vi "CCD Example.vi"(0 "exposure time [ms]":i32=120, 9 "roiConfig":T1={"ROI-index"=1, "xOrigin"=0, "yOrigin"=0, "xSize"=1024, "ySize"=256, "xBin"=1, "yBin"=256}, 11 "error in":errorcluster) -> (4 "ExposureTime [ms]":i32, 6 "device is open?":bool, 13 "chip size, x":i32, 14 "chip size, y":i32, 15 "error out":errorcluster)   [LabVIEW 2023, in "Examples.lvlib"]
doc: "Example for a CCD spectrum acquisition."
uses:
  Examples.lvlib
  Classes/CCD/CCD.lvclass
panel:
  # "Connector Pane"
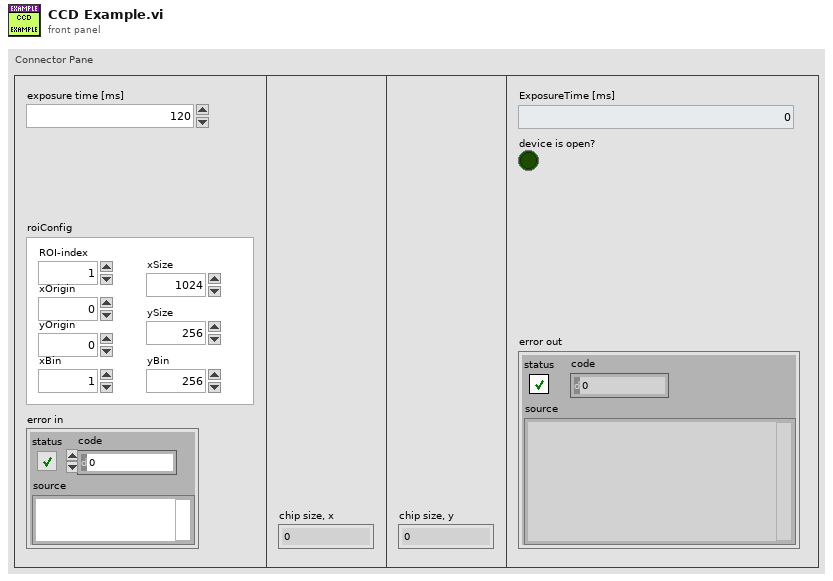
[diagram p1: front panel]
types:
  T1 = cluster{"ROI-index":i32, "xOrigin":i32, "yOrigin":i32, "xSize":i32, "ySize":i32, "xBin":i32, "yBin":i32}
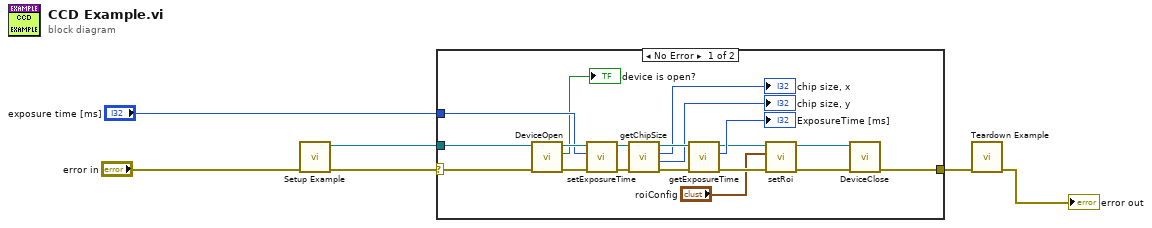
[diagram p0: block diagram]
diagram:
  n1 = call "Setup Example.vi"("error in (no error)"="error in") -> ("error out"=w4:errorcluster, "CCD out"=w3:refnum<class "CCD.lvclass">)  [unwired: 8 in, 1 out]
  n2 = case shown="No Error" w4 {
    selector: w4 -> [w25 w26]
    tunnel: [w19 w26] -> w2
    tunnel: "exposure time [ms]" -> [w20 _]
    tunnel: w3 -> [w7 _]
    frame No Error {
      n3 = call-dynamic "DeviceOpen.vi"("error in (no error)"=w25, "CCD in"=w7) -> ("error out"=w24:errorcluster, "device is open?"=→"device is open?":bool, "CCD out"=w22:refnum<class "CCD.lvclass">)  [unwired: 6 in, 1 out]
      n4 = call "setExposureTime.vi"("error in (no error)"=w24, "exposure time [ms] or [us]"=w20, "CCD in"=w22) -> ("error out"=w23:errorcluster, "CCD out"=w21:refnum<class "CCD.lvclass">)  [unwired: 5 in, 2 out]
      n5 = call-dynamic "getChipSize.vi"("error in (no error)"=w23, "CCD in"=w21) -> ("error out"=w17:errorcluster, "chip size, y"=→"chip size, y":i32, "chip size, x"=→"chip size, x":i32, "CCD out"=w18:refnum<class "CCD.lvclass">)  [unwired: 6 in]
      n6 = call "getExposureTime.vi"("error in (no error)"=w17, "CCD in"=w18) -> ("error out"=w10:errorcluster, "time [ms] or [us]"=→"ExposureTime [ms]":i32, "CCD out"=w12:refnum<class "CCD.lvclass">)  [unwired: 7 in]
      n7 = call "setRoi.vi"("error in (no error)"=w10, "roiConfig"="roiConfig", "CCD in"=w12) -> ("error out"=w9:errorcluster, "CCD out"=w11:refnum<class "CCD.lvclass">)  [unwired: 5 in, 2 out]
      n8 = call-dynamic "DeviceClose.vi"("error in (no error)"=w9, "CCD in"=w11) -> ("error out"=w19:errorcluster)  [unwired: 5 in, 4 out]
    }
    frame Error {
    }
  }
  n9 = call "Teardown Example.vi"("error in (no error)"=w2) -> ("error out"=→"error out":errorcluster)  [unwired: 10 in]
